vi "01地址状态值.vi"(0 "unsigned byte array":u8[](array[numeric]) format="%x") -> (5 "E2初始化完成":bool, 6 "电流校正完成":bool, 7 "启停状态":bool, 8 "转矩模式":bool, 9 "电流校正":bool, 10 "转速模式":bool)   [LabVIEW 2012]
panel:
  out "均有效":bool
  out "DEF有效":bool
  out "ABC有效":bool
  out "自动选择":bool
  out "开环模式":bool
  out "置位复位":bool
  out "数值 2":u32
  out "数值":u32
  out "霍尔位置":u32
  out "mode":u32
  out "数组":bool[](array[boolean])
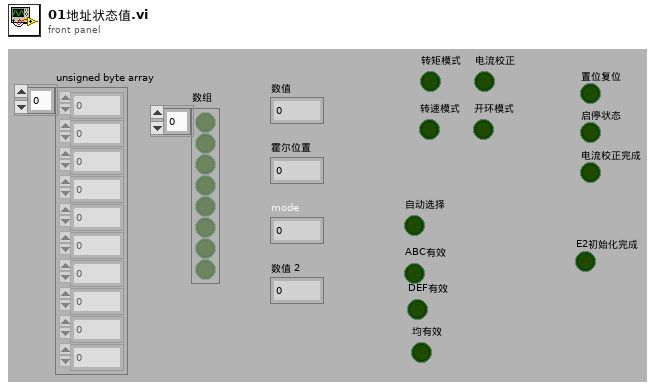
[diagram p1: front panel]
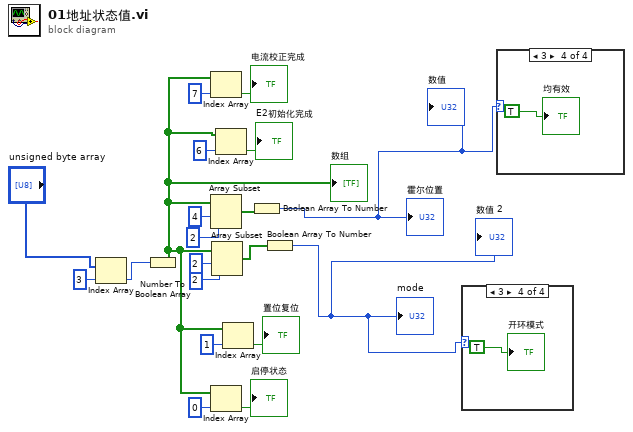
[diagram p0: block diagram]
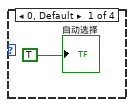
[diagram p2: hidden frame]
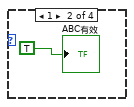
[diagram p3: hidden frame]
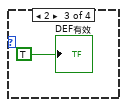
[diagram p4: hidden frame]
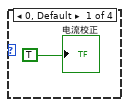
[diagram p5: hidden frame]
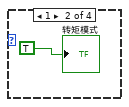
[diagram p6: hidden frame]
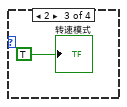
[diagram p7: hidden frame]
diagram:
  n1 = Index Array(array="unsigned byte array", index=3 ("索引")) -> (element=w14:u8)
  n2 = Number To Boolean Array(number=w14) -> (Boolean array=w4:bool[])
  "数组" <- w4
  n3 = Index Array(array=w4, index=7 ("索引")) -> (element=→"电流校正完成":bool)
  n4 = Array Subset(array=w4, index=4 ("索引"), length=2 ("长度")) -> (w20:bool[])
  n5 = Index Array(array=w4, index=0 ("索引")) -> (element=→"启停状态":bool)
  n6 = Array Subset(array=w4, index=2 ("索引"), length=2 ("长度")) -> (w17:bool[])
  n7 = Index Array(array=w4, index=6 ("索引")) -> (element=→"E2初始化完成":bool)
  n8 = Index Array(array=w4, index=1 ("索引")) -> (element=→"置位复位":bool)
  n9 = Boolean Array To Number(Boolean array=w20) -> (number=w2:u32)
  "霍尔位置" <- w2
  "数值" <- w2
  n10 = Boolean Array To Number(Boolean array=w17) -> (number=w3:u32)
  "mode" <- w3
  "数值 2" <- w3
  n11 = case shown="3" w3 {
    frame 0, Default {
      "电流校正" <- TRUE
    }
    frame 1 {
      "转矩模式" <- TRUE
    }
    frame 2 {
      "转速模式" <- TRUE
    }
    frame 3 {
      "开环模式" <- TRUE
    }
  }
  n12 = case shown="3" w2 {
    frame 0, Default {
      "自动选择" <- TRUE
    }
    frame 1 {
      "ABC有效" <- TRUE
    }
    frame 2 {
      "DEF有效" <- TRUE
    }
    frame 3 {
      "均有效" <- TRUE
    }
  }
